vi "live view D03.vi"() -> ()   [LabVIEW 2019, in "D03.lvlib"]
uses:
  D03.lvlib
  <vilib>/userDefined/High Color/IMAQdx.ctl
  <vilib>/vision/Image Controls.llb/IMAQ Image.ctl
  <vilib>/measure/mamon.llb/Trigger Detection for 1 Channel.vi
  <vilib>/measure/NI_MAPro.lvlib
  Calibration Lib.lvlib
  database.lvlib
  <vilib>/vision/driver/NI_Vision_Acquisition_Software.lvlib
panel:
  out "Error out":errorcluster
  in  "Save Button":bool
  in  "Calib IMQ Num":u16(ring) items=["First IMQ", "Second IMQ", "Third IMQ"]
  in  "Verify Calibration1 D03":bool caption="capture grab"
  in  "snapshot":bool
  out "error prj03":errorcluster
  in  "Verify Calibration D03":bool caption="capture grab"
  in  "Close":bool
  in  "Method 2 save D03":bool caption="capture grab"
  in  "Method 1 Save D03":bool caption="Saving txt"
  out "Average Result":string="Average Result"
  out ">18  A":dbl(slide)=1.0 caption=">18 mm" scale=0.0..100.0
  out "16-18  A":dbl(slide)=1.0 caption="16-18 mm" scale=0.0..100.0
  out "14-16  A":dbl(slide)=1.0 caption="14-16 mm" scale=0.0..100.0
  out "12.5-14 A":dbl(slide)=1.0 caption="12.5-14 mm" scale=0.0..100.0
  out "10-12.5  A":dbl(slide)=1.0 caption="10-12.5 mm" scale=0.0..100.0 scale format="%#_4f"
  out "8-10  A":dbl(slide)=1.0 caption="8-10 mm" scale=0.0..100.0
  out "6.3-8  A":dbl(slide)=1.0 caption="6.3-8 mm" scale=0.0..100.0
  out "<6.3  A":dbl(slide)=1.0 caption="<6.3 mm" scale=0.0..100.0
  out "Live Result":string="Live Result"
  out ">18  L":dbl(slide)=1.0 caption=">18 mm" scale=0.0..100.0
  out "Live View":T1(plugin-control) caption="Disc 26"
  out "16-18  L":dbl(slide)=1.0 caption="16-18 mm" scale=0.0..100.0
  out "14-16  L":dbl(slide)=1.0 caption="14-16 mm" scale=0.0..100.0
  out "12.5-14 L":dbl(slide)=1.0 caption="12.5-14 mm" scale=0.0..100.0
  out "10-12.5  L":dbl(slide)=1.0 caption="10-12.5 mm" scale=0.0..100.0 scale format="%#_4f"
  out "8-10  L":dbl(slide)=1.0 caption="8-10 mm" scale=0.0..100.0
  out "6.3-8  L":dbl(slide)=1.0 caption="6.3-8 mm" scale=0.0..100.0
  out "<6.3  L":dbl(slide)=1.0 caption="<6.3 mm" scale=0.0..100.0
  out "disc name":string="Live Info Disc 03"
  out "dsgs":string="DSGS"
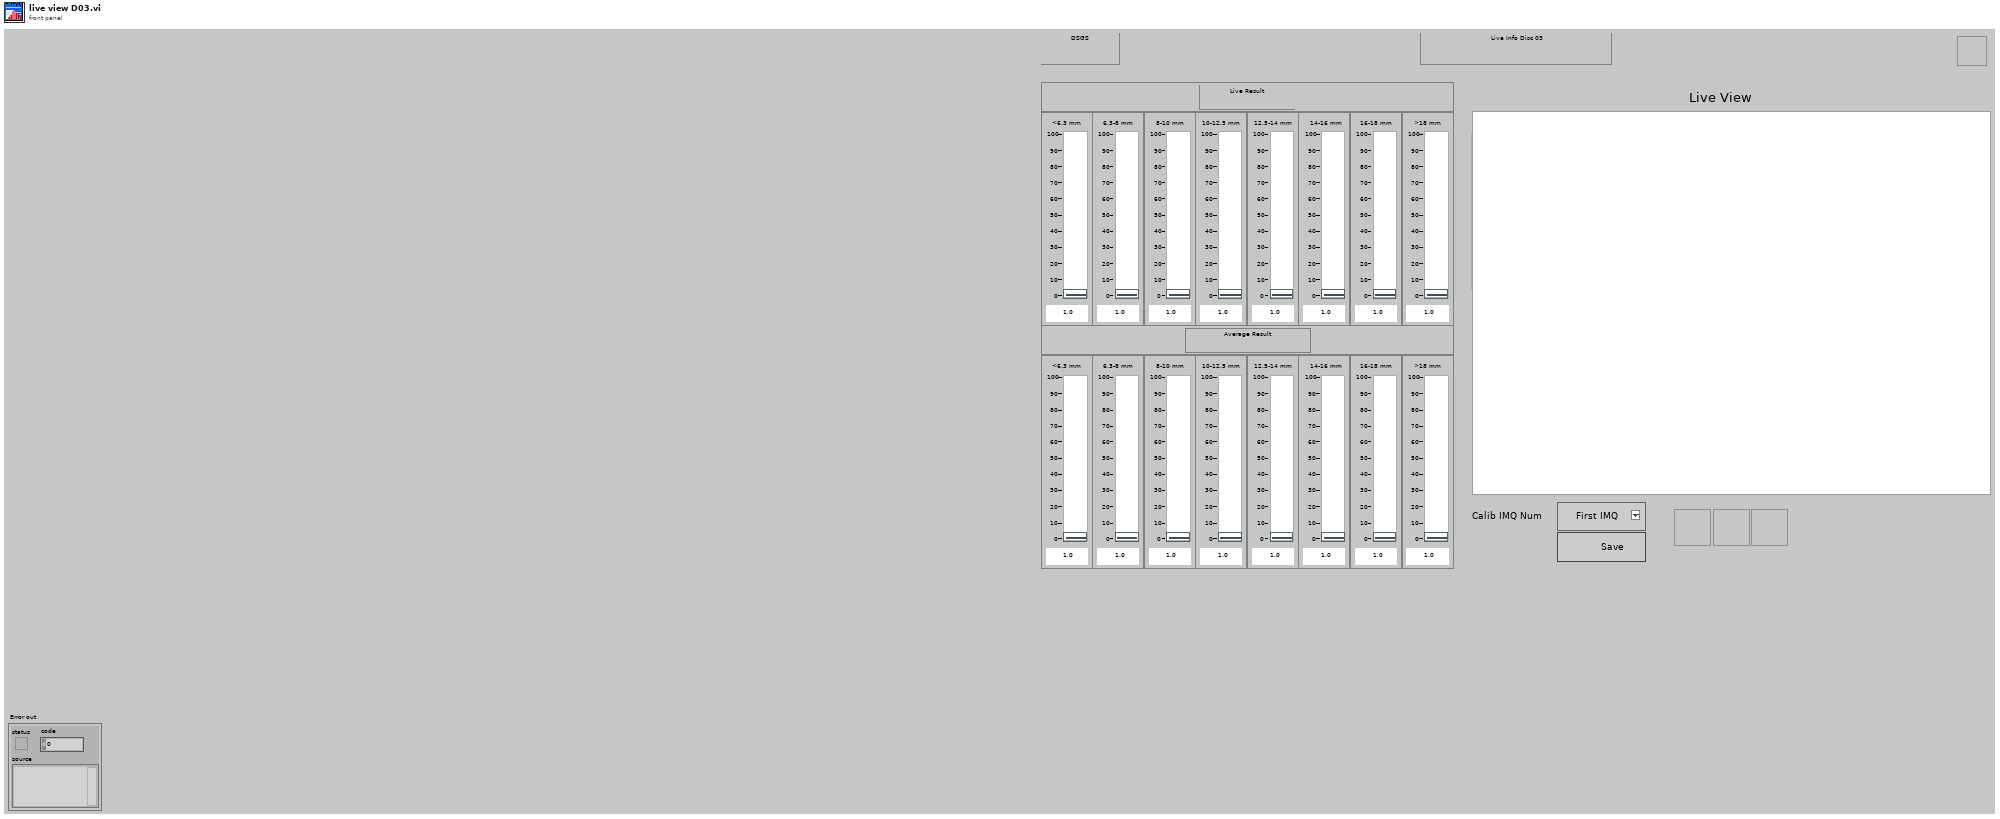
[diagram p1: front panel]
types:
  T1 = typedef "IMAQ Image.ctl" = refnum<image>
  T2 = typedef "IMAQdx.ctl" = refnum<k21>
  T3 = enum8{"Enabled", "Disabled", "Disabled and Grayed Out"}
  T4 = cluster{"date/time string":string, "date/time string":string, string, "Value":dbl, "Value":dbl, "Value":dbl, "Value":dbl, "Value":dbl, "Value":dbl, "Value":dbl, "Value":dbl}
  T5 = cluster{"date/time string":string, "date/time string":string, "time format string (%c)":string, "spreadsheet string":string, "spreadsheet string":string}
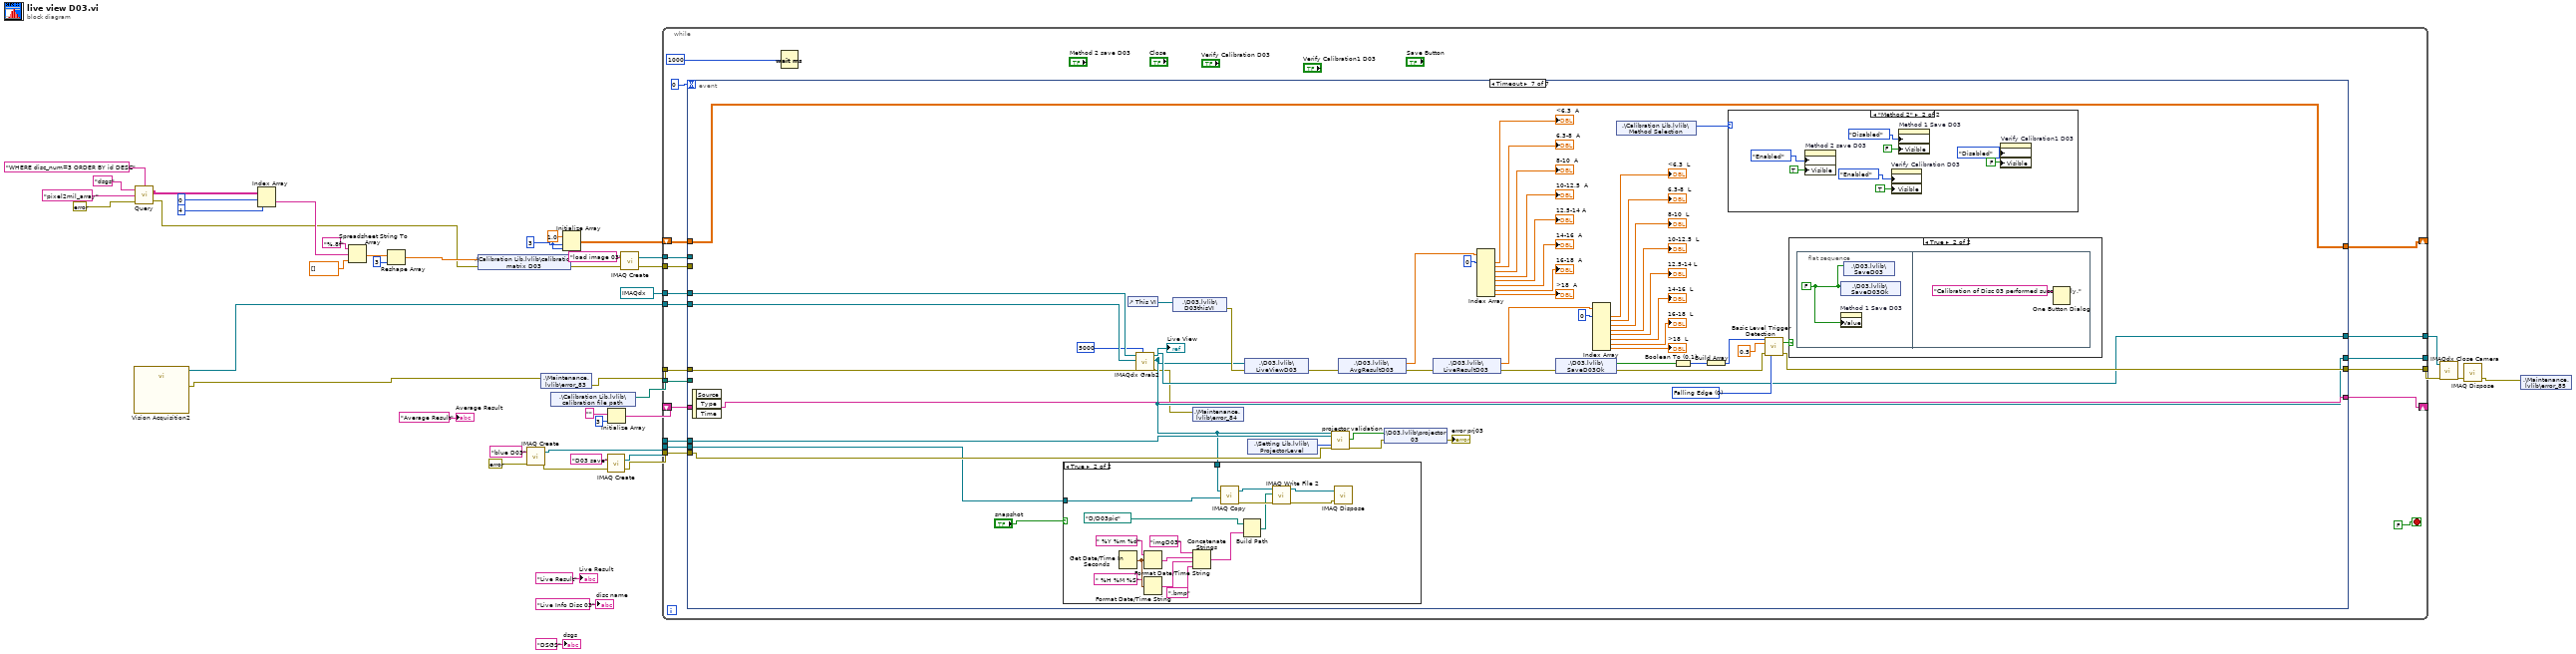
[diagram p0: block diagram]
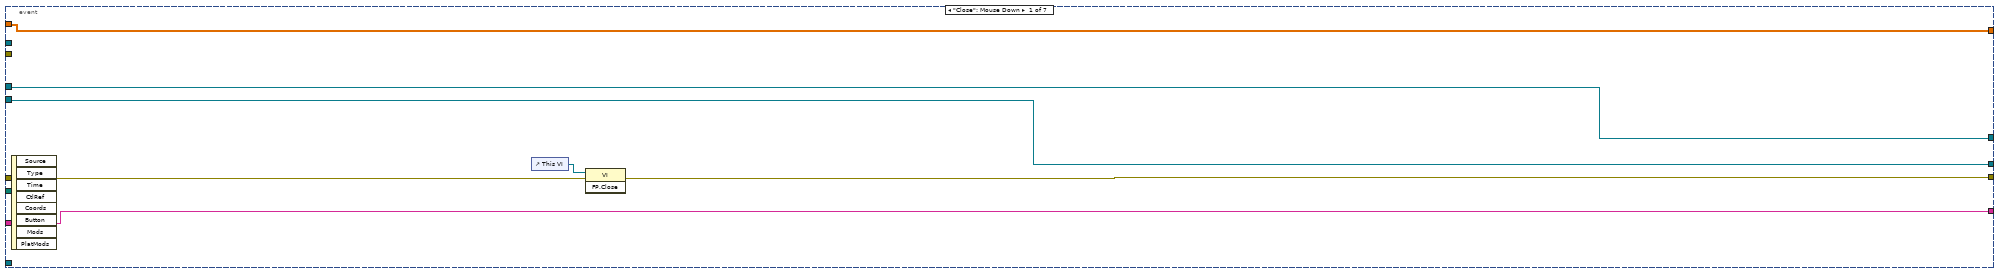
[diagram p2: hidden frame]
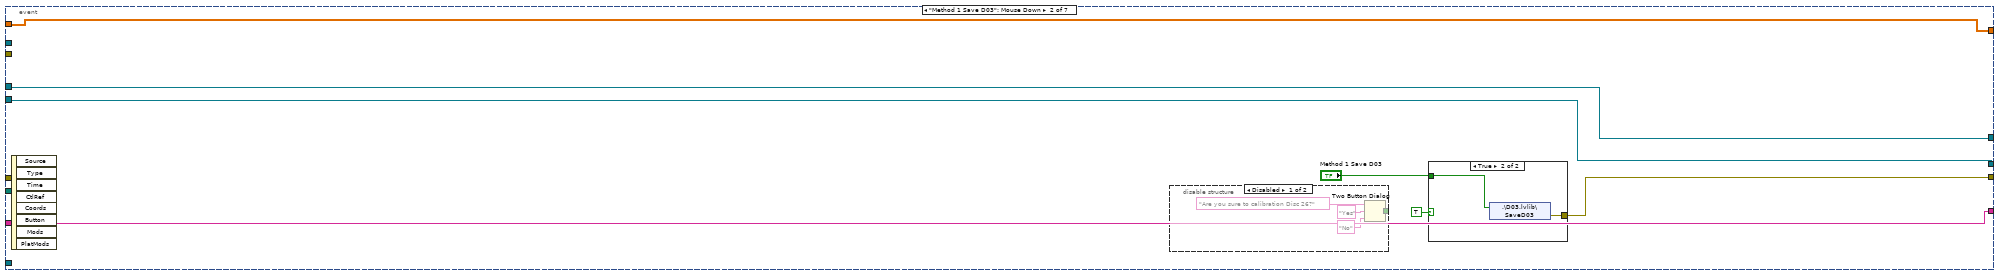
[diagram p3: hidden frame]
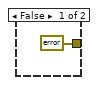
[diagram p5: hidden frame]
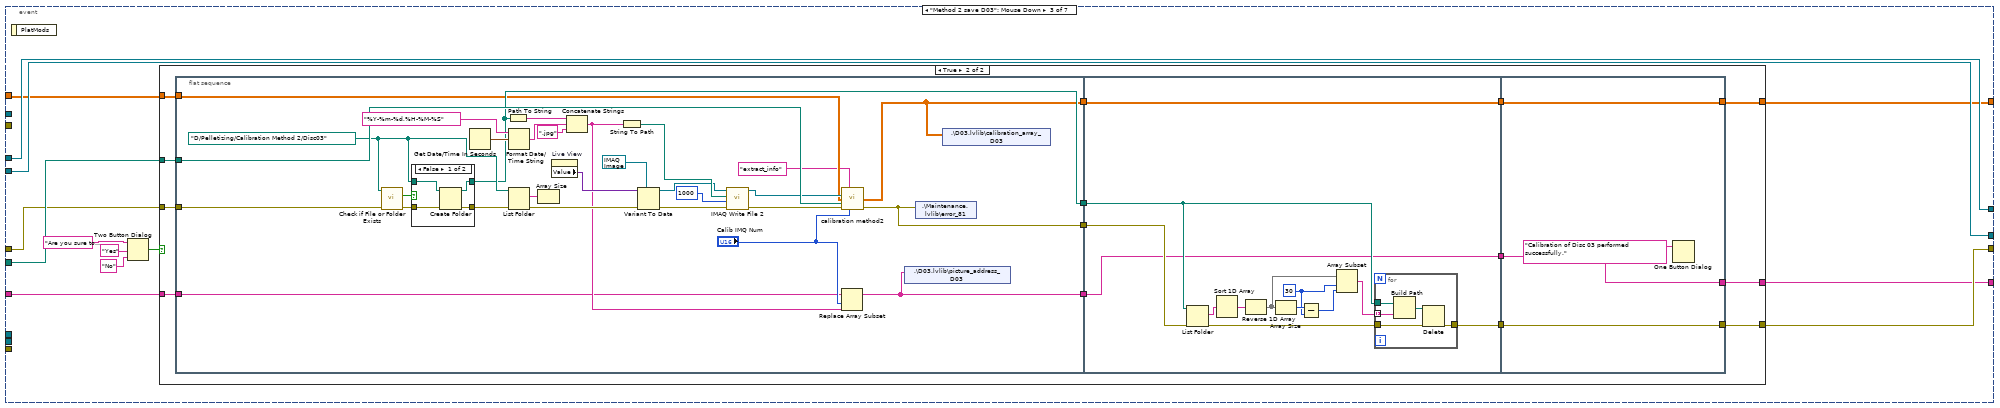
[diagram p6: hidden frame]
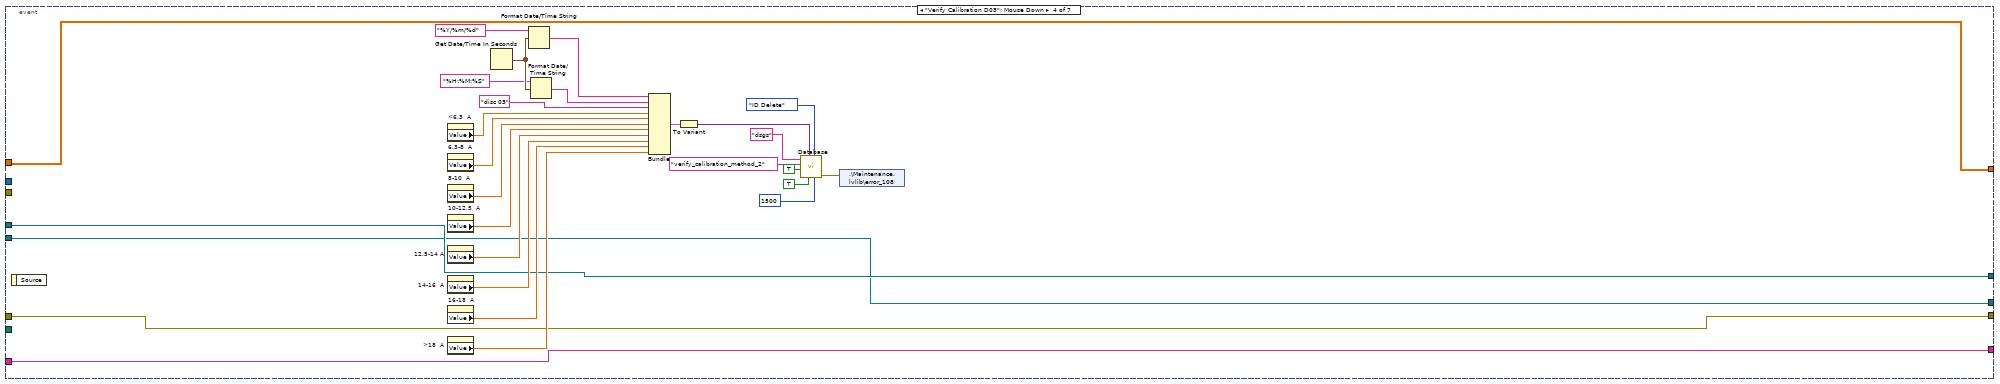
[diagram p9: hidden frame]
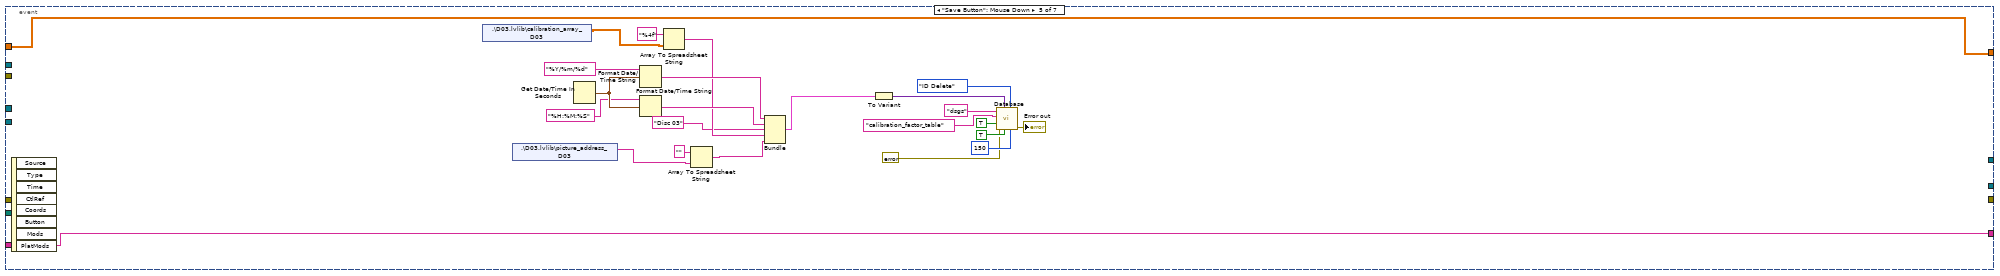
[diagram p10: hidden frame]
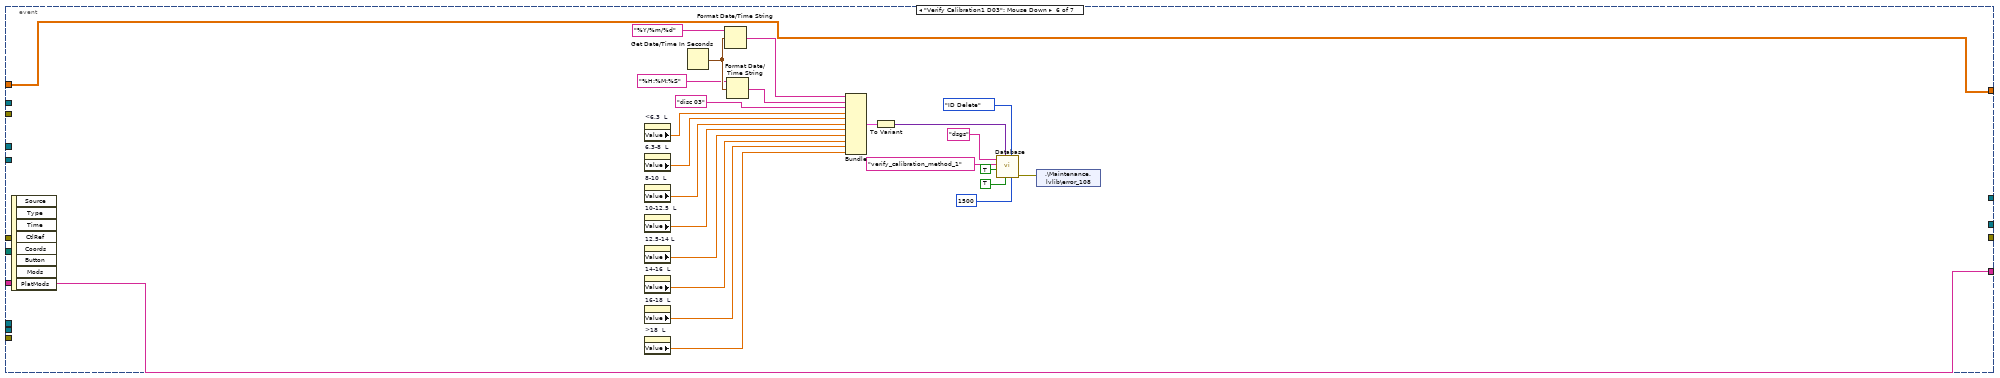
[diagram p11: hidden frame]
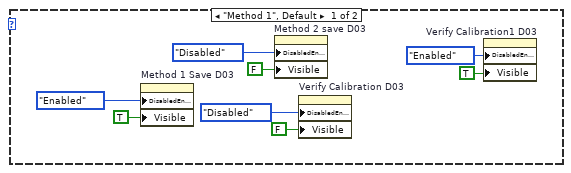
[diagram p13: hidden frame]
diagram:
  w13 = 3 ("dimension size")
  n1 = call "Vision Acquisition2"() -> ("Image Out"=w2:T1, "error out"=w1:errorcluster)  [unwired: 25 in, 1 out]
  n2 = call "Query.vi"("Condition"="WHERE disc_num=3 ORDER BY id DESC", "Error in"=errorcluster {"status"=FALSE, "code"=0, "source"=""}, "Table Name"="pixel2mil_array", "Connection Name"="dsgs") -> ("Error out"=w5:errorcluster, "data"=w8:string[][])
  n3 = Index Array(array=w8, index (row)=0, index (col)=4 ("disabled index (col)")) -> (element=w6:string)
  n4 = Spreadsheet String To Array(format string="%.8f", spreadsheet string=w6, array type (2D Dbl)=sgl[] []) -> (array=w26:sgl[])  [unwired: 1 in]
  n5 = Reshape Array(w26, 3 ("dimension size")) -> (w23:sgl[])
  n6 = shared-variable ".\\Calibration Lib.lvlib\\calibration matrix D03"(w23, error in=w5) -> (error out=w22:errorcluster)
  n7 = call "IMAQ Create"("Image Name"="blue D03", "error in (no error)"=errorcluster {"status"=FALSE, "code"=0, "source"=""}) -> ("New Image"=w20:T1, "error out"=w18:errorcluster)  [unwired: 3 in]
  n8 = shared-variable ".\\Maintenance.lvlib\\error_83"(w1) -> (error out=w35:errorcluster)  [unwired: 1 in]
  n9 = shared-variable ".\\Calibration Lib.lvlib\\calibration file path"() -> (w36:path)  [unwired: 1 in, 1 out]
  n10 = Initialize Array(1.0 ("element"), w13, w13) -> (w12:dbl[][])
  n11 = call "IMAQ Create"("Image Name"="D03 save", "error in (no error)"=w18) -> ("New Image"=w15:T1, "error out"=w17:errorcluster)  [unwired: 3 in]
  n12 = Initialize Array("", 3 ("dimension size")) -> (w9:string[])
  n13 = call "IMAQ Create"("Image Name"="load image 03", "error in (no error)"=w22) -> ("New Image"=w32:T1, "error out"=w33:errorcluster)  [unwired: 3 in]
  n14 = while {
    tunnel: w36 -> [w61]
    tunnel: w35 -> [w60]
    tunnel: w2 -> [w58]
    tunnel: [w57] -> w40
    tunnel: [w56] -> _
    tunnel: T2 "cam1" ("Session In") -> [w55]
    tunnel: [w54] -> w37
    tunnel: w33 -> [w53]
    tunnel: w32 -> [w52]
    tunnel: w20 -> [w51]
    tunnel: w17 -> [w50]
    tunnel: w15 -> [w49]
    shift-right: [w47] -> _
    shift-left: w12 -> [w48]
    shift-right: [w45] -> _
    shift-left: w9 -> [w46]
    stop <- FALSE stop-if-true
    n15 = event shown="[6] Timeout" {
      selector: _ -> [_ _ _ _ _ _ _]
      dyn-events: _ -> [_ _ _ _ _ _ _]
      timeout: 0 -> [_ _ _ _ _ _ _]
      tunnel: w61 -> [_ _ w97 _ _ _ _]
      tunnel: [w69 w77 w93 w179 _ _ w268] -> w57
      tunnel: w60 -> [w68 _ w96 w179 _ _ w256]
      tunnel: w58 -> [w67 w76 w95 w177 _ _ w251]
      tunnel: [w67 w76 w95 w177 _ _ w253] -> w56
      tunnel: w55 -> [w66 w75 w94 w178 _ _ w255]
      tunnel: [w66 w75 w94 w178 _ _ w254] -> w54
      tunnel: w53 -> [_ _ _ _ _ _ _]
      tunnel: w52 -> [_ _ _ _ _ _ _]
      tunnel: w51 -> [_ _ _ _ _ _ w266]
      tunnel: w50 -> [_ _ _ _ _ _ w262]
      tunnel: w49 -> [_ _ _ _ _ _ w259]
      tunnel: w48 -> [w65 w72 w88 w174 w203 w226 w258]
      tunnel: [w65 w72 w87 w174 w203 w226 w258] -> w47
      tunnel: w46 -> [w64 w71 w86 w173 w202 w225 w257]
      tunnel: [w64 w71 w85 w173 w202 w225 w257] -> w45
      event "Close": Mouse Down {
        n16 = event-data() -> ()  [unwired: 1 in, 8 out]
        n17 = control-ref of="This VI"() -> (w70:refnum<vi>)
        n18 = invoke class="VI" method="FP.Close"(reference=w70, error in=w68) -> (error out=w69:errorcluster)  [unwired: 1 in, 2 out]
      }
      event "Method 1 Save D03": Mouse Down {
        n19 = event-data() -> ()  [unwired: 1 in, 8 out]
        n20 = disable-structure shown="Disabled" {
          disable-tunnel: [w78 _] -> _
          frame Disabled {
            n21 = Two Button Dialog(message="Are you sure to calibration Disc 26?", 1:"No" ("F button name (\"Cancel\")"), 2:"Yes" ("T button name (\"OK\")")) -> (T button?=w78:bool)
          }
          frame Enabled {
          }
        }
        n22 = case shown="True" TRUE {
          tunnel: [errorcluster {"status"=FALSE, "code"=0, "source"=""} ("error IO") w84] -> w77
          tunnel: "Method 1 Save D03" -> [_ w83]
          frame False {
          }
          frame True {
            n23 = shared-variable ".\\D03.lvlib\\SaveD03"(w83) -> (error out=w84:errorcluster)  [unwired: 1 in]
          }
        }
      }
      event "Method 2 save D03": Mouse Down {
        n24 = event-data() -> ()  [unwired: 1 in, 1 out]
        n25 = Two Button Dialog(message="Are you sure to calibration Disc 26?", 1:"No" ("F button name (\"Cancel\")"), 2:"Yes" ("T button name (\"OK\")")) -> (T button?=w89:bool)
        n26 = case shown="True" w89 {
          tunnel: w97 -> [_ w113]
          tunnel: w96 -> [w100 w112]
          tunnel: [w100 w111] -> w93
          tunnel: w88 -> [w99 w109]
          tunnel: [w99 w106] -> w87
          tunnel: w86 -> [w98 w105]
          tunnel: [w98 w102] -> w85
          frame False {
          }
          frame True {
            n27 = flat-sequence {
              tunnel: w112 -> [w133]
              tunnel: w113 -> [w144]
              tunnel: [w126] -> w114
              tunnel: w109 -> [w123]
              tunnel: [w122] -> w107
              tunnel: w105 -> [w117]
              tunnel: [w116] -> w103
              tunnel: [w115] -> w101
              tunnel: [w154] -> w110
              tunnel: [w152] -> w108
              tunnel: [w151] -> w104
              tunnel: w101 -> [w155]
              tunnel: w103 -> [w151]
              tunnel: w107 -> [w152]
              tunnel: w114 -> [w156]
              tunnel: [w172] -> w111
              tunnel: w110 -> [w172]
              tunnel: [w170] -> w106
              tunnel: w108 -> [w170]
              tunnel: [w169] -> w102
              tunnel: w104 -> [w169]
              frame #0 {
                w127 = path "D:/Pelletizing/Calibration Method 2/Disc03" ("path")
                n28 = call <vilib>:"Check if File or Folder Exists.vi"("error in (no error)"=w133, "path"=w127) -> ("error out"=w134:errorcluster, "file or folder exists?"=w135:bool)  [unwired: 7 in, 1 out]
                n29 = case shown="False" w135 {
                  tunnel: [w146 w150] -> w126
                  tunnel: w127 -> [w148 w150]
                  tunnel: w134 -> [w147 w149]
                  tunnel: [w145 w149] -> w129
                  frame False {
                    n30 = Create Folder(path (use dialog)=w148, error in=w147) -> (created path=w146:path, error out=w145:errorcluster)  [unwired: 1 in, 1 out]
                  }
                  frame True {
                  }
                }
                n31 = Get Date/Time In Seconds() -> (seconds since 1Jan1904=w139:timestamp)
                n32 = Path To String(path=w126) -> (string=w131:string)
                n33 = Format Date/Time String(time format string (%c)="%Y-%m-%d,%H-%M-%S", seconds (now)=w139) -> (date/time string=w137:string)  [unwired: 1 in]
                n34 = List Folder(path=w127, error in=w129) -> (filenames=w130:string[], error out=w128:errorcluster)  [unwired: 2 in, 2 out]
                n35 = Array Size(array=w130) -> ()  [unwired: 1 out]
                n36 = property on="Live View" class="ImageControl"() -> ("Value"=w143:variant)  [unwired: 2 in, 2 out]
                n37 = Concatenate Strings(w131, w137, ".jpg" ("string")) -> (w119:string)
                n38 = String To Path(string=w119) -> (path=w132:path)
                n39 = Variant To Data(error in=w128, type=T1 refnum ("New Image"), Variant=w143) -> (data=w124:T1, error out=w140:errorcluster)
                n40 = call-poly "IMAQ Write File 2"("error in (no error)"=w140, "Image Quality"=u32 1000, "File Path"=w132, "Image"=w124) -> ("error out"=w121:errorcluster, "Image Out (duplicate)"=w125:T1)  [unwired: 6 in]
                n41 = Replace Array Subset(array=w117, new element=w119, index="Calib IMQ Num") -> (w116:string[])
                n42 = call "calibration method2.vi"("function name"="extract_info", "Image IN"=w125, "initialize matrix"=w123, "module path"=w144, "error in"=w121, "snap number"="Calib IMQ Num") -> ("calibration matrix"=w122:dbl[][], "error out"=w115:errorcluster)  [unwired: 8 in]
                n43 = shared-variable ".\\D03.lvlib\\picture_address_D03"(w116) -> ()  [unwired: 1 in, 1 out]
                n44 = shared-variable ".\\Maintenance.lvlib\\error_81"(w115) -> ()  [unwired: 1 in, 1 out]
                n45 = shared-variable ".\\D03.lvlib\\calibration_array_D03"(w122) -> ()  [unwired: 1 in, 1 out]
              }
              frame #1 {
                w157 = 30 ("index")
                n46 = List Folder(path=w156, error in=w155) -> (filenames=w163:string[], error out=w153:errorcluster)  [unwired: 2 in, 2 out]
                n47 = Sort 1D Array(array=w163) -> (sorted array=w162:string[])
                n48 = Reverse 1D Array(array=w162) -> (reversed array=w161:string[])
                n49 = Array Size(array=w161) -> (size(s)=w160:i32)
                n50 = Subtract(x=w160, y=w157) -> (x-y=w159:i32)
                n51 = Array Subset(array=w161, index=w157, length=w159) -> (w158:string[])
                n52 = for {
                  tunnel: w158 -> [w167] mode=indexing
                  tunnel: w156 -> [w168]
                  tunnel: [w165] -> w154
                  tunnel: w153 -> [w164]
                  n53 = Build Path(base path=w168, name or relative path=w167) -> (appended path=w166:path)
                  n54 = Delete(path (use dialog)=w166, error in=w164) -> (error out=w165:errorcluster)  [unwired: 3 in, 2 out]
                }
              }
              frame #2 {
                n55 = One Button Dialog(message="Calibration of Disc 03 performed successfully.") -> ()  [unwired: 1 in, 1 out]
              }
            }
          }
        }
      }
      event "Verify Calibration D03": Mouse Down {
        n56 = event-data() -> ()  [unwired: 1 in, 1 out]
        n57 = property on="<6.3  A" class="Slide (strict)"() -> ("Value"=w194:dbl)  [unwired: 2 in, 2 out]
        n58 = property on="6.3-8  A" class="Slide (strict)"() -> ("Value"=w193:dbl)  [unwired: 2 in, 2 out]
        n59 = property on="8-10  A" class="Slide (strict)"() -> ("Value"=w192:dbl)  [unwired: 2 in, 2 out]
        n60 = property on="10-12.5  A" class="Slide (strict)"() -> ("Value"=w191:dbl)  [unwired: 2 in, 2 out]
        n61 = property on="12.5-14 A" class="Slide (strict)"() -> ("Value"=w190:dbl)  [unwired: 2 in, 2 out]
        n62 = property on="14-16  A" class="Slide (strict)"() -> ("Value"=w189:dbl)  [unwired: 2 in, 2 out]
        n63 = property on="16-18  A" class="Slide (strict)"() -> ("Value"=w188:dbl)  [unwired: 2 in, 2 out]
        n64 = property on=">18  A" class="Slide (strict)"() -> ("Value"=w187:dbl)  [unwired: 2 in, 2 out]
        n65 = Get Date/Time In Seconds() -> (seconds since 1Jan1904=w199:timestamp)
        n66 = Format Date/Time String(time format string (%c)="%Y/%m/%d", seconds (now)=w199) -> (date/time string=w197:string)  [unwired: 1 in]
        n67 = Format Date/Time String(time format string (%c)="%H:%M:%S", seconds (now)=w199) -> (date/time string=w196:string)  [unwired: 1 in]
        n68 = Bundle("date/time string"=w197, "date/time string"=w196, "disc 03", "Value"=w194, "Value"=w193, "Value"=w192, "Value"=w191, "Value"=w190, "Value"=w189, "Value"=w188, "Value"=w187) -> (w186:T4)  [unwired: 1 in]
        n69 = To Variant(anything=w186) -> (Variant=w185:variant)
        n70 = call "Database.vi"("Maximum Row"=1500, "Enum"=enum16{"ID Delete", "Time Delete"}."ID Delete", "Delete row?"=TRUE, "Data"=w185, "Auto Increment ID?"=TRUE, "Table"="verify_calibration_method_2", "Connection"="dsgs") -> ("Error out"=w180:errorcluster)  [unwired: 4 in]
        n71 = shared-variable ".\\Maintenance.lvlib\\error_108"(w180) -> ()  [unwired: 1 in, 1 out]
      }
      event "Save Button": Mouse Down {
        n72 = event-data() -> ()  [unwired: 1 in, 8 out]
        n73 = shared-variable ".\\D03.lvlib\\calibration_array_D03"() -> (w204:dbl[][])  [unwired: 1 in, 1 out]
        n74 = shared-variable ".\\D03.lvlib\\picture_address_D03"() -> (w206:string[])  [unwired: 1 in, 1 out]
        n75 = Get Date/Time In Seconds() -> (seconds since 1Jan1904=w213:timestamp)
        n76 = Format Date/Time String(time format string (%c)="%Y/%m/%d", seconds (now)=w213) -> (date/time string=w214:string)  [unwired: 1 in]
        n77 = Format Date/Time String(time format string (%c)="%H:%M:%S", seconds (now)=w213) -> (date/time string=w212:string)  [unwired: 1 in]
        n78 = Array To Spreadsheet String(array=w204, 3:"%4f" ("format string")) -> (spreadsheet string=w208:string)  [unwired: 1 in]
        n79 = Array To Spreadsheet String(array=w206, 3:"" ("format string")) -> (spreadsheet string=w205:string)  [unwired: 1 in]
        n80 = Bundle("date/time string"=w214, "date/time string"=w212, "time format string (%c)"="Disc 03", "spreadsheet string"=w208, "spreadsheet string"=w205) -> (w217:T5)  [unwired: 1 in]
        n81 = To Variant(anything=w217) -> (Variant=w224:variant)
        n82 = call "Database.vi"("Maximum Row"=150, "Enum"=enum16{"ID Delete", "Time Delete"}."ID Delete", "Delete row?"=TRUE, "Data"=w224, "Error in"=errorcluster {"status"=FALSE, "code"=0, "source"=""}, "Auto Increment ID?"=TRUE, "Table"="calibration_factor_table", "Connection"="dsgs") -> ("Error out"=→"Error out":errorcluster)  [unwired: 3 in]
      }
      event "Verify Calibration1 D03": Mouse Down {
        n83 = event-data() -> ()  [unwired: 1 in, 8 out]
        n84 = property on="<6.3  L" class="Slide (strict)"() -> ("Value"=w243:dbl)  [unwired: 2 in, 2 out]
        n85 = property on="6.3-8  L" class="Slide (strict)"() -> ("Value"=w242:dbl)  [unwired: 2 in, 2 out]
        n86 = property on="8-10  L" class="Slide (strict)"() -> ("Value"=w241:dbl)  [unwired: 2 in, 2 out]
        n87 = property on="10-12.5  L" class="Slide (strict)"() -> ("Value"=w240:dbl)  [unwired: 2 in, 2 out]
        n88 = property on="12.5-14 L" class="Slide (strict)"() -> ("Value"=w239:dbl)  [unwired: 2 in, 2 out]
        n89 = property on="14-16  L" class="Slide (strict)"() -> ("Value"=w238:dbl)  [unwired: 2 in, 2 out]
        n90 = property on="16-18  L" class="Slide (strict)"() -> ("Value"=w237:dbl)  [unwired: 2 in, 2 out]
        n91 = property on=">18  L" class="Slide (strict)"() -> ("Value"=w236:dbl)  [unwired: 2 in, 2 out]
        n92 = Get Date/Time In Seconds() -> (seconds since 1Jan1904=w248:timestamp)
        n93 = Format Date/Time String(time format string (%c)="%Y/%m/%d", seconds (now)=w248) -> (date/time string=w246:string)  [unwired: 1 in]
        n94 = Format Date/Time String(time format string (%c)="%H:%M:%S", seconds (now)=w248) -> (date/time string=w245:string)  [unwired: 1 in]
        n95 = Bundle("date/time string"=w246, "date/time string"=w245, "disc 03", "Value"=w243, "Value"=w242, "Value"=w241, "Value"=w240, "Value"=w239, "Value"=w238, "Value"=w237, "Value"=w236) -> (w235:T4)  [unwired: 1 in]
        n96 = To Variant(anything=w235) -> (Variant=w234:variant)
        n97 = call "Database.vi"("Maximum Row"=1500, "Enum"=enum16{"ID Delete", "Time Delete"}."ID Delete", "Delete row?"=TRUE, "Data"=w234, "Auto Increment ID?"=TRUE, "Table"="verify_calibration_method_1", "Connection"="dsgs") -> ("Error out"=w229:errorcluster)  [unwired: 4 in]
        n98 = shared-variable ".\\Maintenance.lvlib\\error_108"(w229) -> ()  [unwired: 1 in, 1 out]
      }
      event Timeout {
        w276 = u16 0 items=["Falling Edge", "Rising Edge"] ("trigger slope")
        n99 = event-data() -> ()  [unwired: 1 in, 3 out]
        n100 = control-ref of="This VI"() -> (w271:refnum<vi>)
        n101 = call <vilib>:"IMAQdx Grab2.vi"("Timeout (ms)"=5000, "error in"=w256, "Image In"=w251, "Session In"=w255) -> ("error out"=w252:errorcluster, "Image Out"=w253:T1, "Session Out"=w254:T2)  [unwired: 4 in, 1 out]
        "Live View" <- w253
        n102 = case shown="True" "snapshot" {
          tunnel: w259 -> [_ w316]
          tunnel: w253 -> [_ w315]
          frame False {
          }
          frame True {
            n103 = Get Date/Time In Seconds() -> (seconds since 1Jan1904=w309:timestamp)
            n104 = Format Date/Time String(time format string (%c)=" %Y %m %d", seconds (now)=w309) -> (date/time string=w305:string)  [unwired: 1 in]
            n105 = Format Date/Time String(time format string (%c)=" %H %M %S", seconds (now)=w309) -> (date/time string=w304:string)  [unwired: 1 in]
            n106 = Concatenate Strings("imgD03" ("string"), w305, w304, ".bmp" ("string")) -> (w302:string)
            n107 = call "IMAQ Copy"("Image Dst"=w316, "Image Src"=w315) -> ("error out"=w313:errorcluster, "Image Dst Out"=w314:T1)  [unwired: 4 in]
            n108 = Build Path(base path=path "D:/D03pic" ("File Path"), name or relative path=w302) -> (appended path=w301:path)
            n109 = call-poly "IMAQ Write File 2"("error in (no error)"=w313, "File Path"=w301, "Image"=w314) -> ("error out"=w311:errorcluster, "Image Out (duplicate)"=w312:T1)  [unwired: 7 in]
            n110 = call "IMAQ Dispose"("Image"=w312, "error in (no error)"=w311) -> ()  [unwired: 4 in, 1 out]
          }
        }
        n111 = shared-variable ".\\D03.lvlib\\D03thisVI"(w271) -> (error out=w267:errorcluster)  [unwired: 1 in]
        n112 = shared-variable ".\\Maintenance.lvlib\\error_84"(w252) -> ()  [unwired: 1 in, 1 out]
        n113 = shared-variable ".\\D03.lvlib\\LiveViewD03"(w253, error in=w267) -> (error out=w270:errorcluster)
        n114 = shared-variable ".\\Setting Lib.lvlib\\ProjectorLevel"() -> (w261:i32)  [unwired: 1 in, 1 out]
        n115 = call "projector validation.vi"("Image Src"=w253, "blue channel"=w266, "on/off level"=w261, "error in (no error)"=w262) -> ("on/off"=w265:bool, "error out"=w264:errorcluster)  [unwired: 14 in]
        n116 = shared-variable ".\\D03.lvlib\\AvgResultD03"(error in=w270) -> (w291:dbl[], error out=w273:errorcluster)
        n117 = shared-variable ".\\D03.lvlib\\projector 03"(w265, error in=w264) -> (error out=→"error prj03":errorcluster)
        n118 = shared-variable ".\\D03.lvlib\\LiveResultD03"(error in=w273) -> (w290:dbl[], error out=w272:errorcluster)
        n119 = Index Array(array=w291, index #1=0 ("index")) -> (element #1=→"<6.3  A":dbl, element #2=→"6.3-8  A":dbl, element #3=→"8-10  A":dbl, element #4=→"10-12.5  A":dbl, element #5=→"12.5-14 A":dbl, element #6=→"14-16  A":dbl, element #7=→"16-18  A":dbl, element #8=→">18  A":dbl)  [unwired: 7 in]
        n120 = shared-variable ".\\D03.lvlib\\SaveD03Ok"(error in=w272) -> (w277:bool, error out=w269:errorcluster)
        n121 = Index Array(array=w290, index #1=0 ("index")) -> (element #1=→"<6.3  L":dbl, element #2=→"6.3-8  L":dbl, element #3=→"8-10  L":dbl, element #4=→"10-12.5  L":dbl, element #5=→"12.5-14 L":dbl, element #6=→"14-16  L":dbl, element #7=→"16-18  L":dbl, element #8=→">18  L":dbl)  [unwired: 7 in]
        n122 = shared-variable ".\\Calibration Lib.lvlib\\Method Selection"() -> (w274:enum32{"Method 1", "Method 2"})  [unwired: 1 in, 1 out]
        n123 = Boolean To (0,1)(Boolean=w277) -> (0, 1=w280:i16)
        n124 = Build Array(w280) -> (w279:i16[])
        n125 = case shown="\"Method 2\"" w274 {
          frame "Method 1", Default {
            n126 = property on="Method 1 Save D03" class="Bool (strict)"("DisabledEnum"=T3."Enabled" ("Disabled"), "Visible"=TRUE) -> ()  [unwired: 2 in, 2 out]
            n127 = property on="Method 2 save D03" class="Bool (strict)"("DisabledEnum"=T3."Disabled" ("Disabled"), "Visible"=FALSE) -> ()  [unwired: 2 in, 2 out]
            n128 = property on="Verify Calibration D03" class="Bool (strict)"("DisabledEnum"=T3."Disabled" ("Disabled"), "Visible"=FALSE) -> ()  [unwired: 2 in, 2 out]
            n129 = property on="Verify Calibration1 D03" class="Bool (strict)"("DisabledEnum"=T3."Enabled" ("Disabled"), "Visible"=TRUE) -> ()  [unwired: 2 in, 2 out]
          }
          frame "Method 2" {
            n130 = property on="Method 2 save D03" class="Bool (strict)"("DisabledEnum"=T3."Enabled" ("Disabled"), "Visible"=TRUE) -> ()  [unwired: 2 in, 2 out]
            n131 = property on="Verify Calibration D03" class="Bool (strict)"("DisabledEnum"=T3."Enabled" ("Disabled"), "Visible"=TRUE) -> ()  [unwired: 2 in, 2 out]
            n132 = property on="Method 1 Save D03" class="Bool (strict)"("DisabledEnum"=T3."Disabled" ("Disabled"), "Visible"=FALSE) -> ()  [unwired: 2 in, 2 out]
            n133 = property on="Verify Calibration1 D03" class="Bool (strict)"("DisabledEnum"=T3."Disabled" ("Disabled"), "Visible"=FALSE) -> ()  [unwired: 2 in, 2 out]
          }
        }
        n134 = call-poly <vilib>:"Basic Level Trigger Detection.vi"("signal in"=w279, "level"=0.5, "error in (no error)"=w269, "trigger slope"=w276) -> ("trigger detected?"=w275:bool, "error out"=w268:errorcluster)  [unwired: 9 in, 1 out]
        n135 = case shown="True" w275 {
          frame False {
          }
          frame True {
            n136 = flat-sequence {
              frame #0 {
                w333 = FALSE
                n137 = shared-variable ".\\D03.lvlib\\SaveD03Ok"(w333) -> ()  [unwired: 1 in, 1 out]
                n138 = property on="Method 1 Save D03" class="Bool (strict)"("Value"=w333) -> ()  [unwired: 2 in, 2 out]
                n139 = shared-variable ".\\D03.lvlib\\SaveD03"(w333) -> ()  [unwired: 1 in, 1 out]
              }
              frame #1 {
                n140 = One Button Dialog(message="Calibration of Disc 03 performed successfully.") -> ()  [unwired: 1 in, 1 out]
              }
            }
          }
        }
      }
    }
    n141 = Wait (ms)(milliseconds to wait=u32 1000) -> ()  [unwired: 1 out]
  }
  n142 = call <vilib>:"IMAQdx Close Camera.vi"("error in"=w40, "Session In"=w37) -> ("error out"=w39:errorcluster)  [unwired: 9 in]
  n143 = call "IMAQ Dispose"("error in (no error)"=w39) -> ("error out"=w3:errorcluster)  [unwired: 5 in]
  n144 = shared-variable ".\\Maintenance.lvlib\\error_85"(w3) -> ()  [unwired: 1 in, 1 out]
  "Live Result" <- "Live Result" ("Live Result")
  "Average Result" <- "Average Result" ("Average Result")
  "disc name" <- "Live Info Disc 03" ("Live Result")
  "dsgs" <- "DSGS" ("Live Result")
